vi "Read 3D Mesh Property Array.vi"(8 "error in (no error)":errorcluster, 11 "3D Mesh.lvclass in":refnum<class "3D Mesh.lvclass">) -> (0 "error out":errorcluster, 2 "3D Mesh Property Array":T1, 3 "3D Mesh.lvclass out":refnum<class "3D Mesh.lvclass">)   [LabVIEW 2020, in "3D Mesh.lvclass"]
uses:
  <vilib>/Math Plots/3D Math Plots/3D Mesh/3D Mesh/3D Mesh.lvclass
  <vilib>/Math Plots/3D Math Plots/3D Mesh/3D Mesh/Typedef/3D Mesh Propery Array.ctl
  <vilib>/Math Plots/3D Math Plots/3D Mesh/3D Mesh/Typedef/3D Mesh Property.ctl
  <vilib>/Math Plots/3D Math Plots/3D Plot/3D Plot/Typedef/Line Type.ctl
  <vilib>/Math Plots/3D Math Plots/3D Plot/3D Plot/Typedef/Color Ramp Cluster.ctl
  <vilib>/Math Plots/3D Math Plots/3D Mesh/3D Mesh/3D Mesh.lvclass/3D Mesh.ctl
  <vilib>/Math Plots/3D Math Plots/3D Plot/3D Plot/3D Plot.lvclass
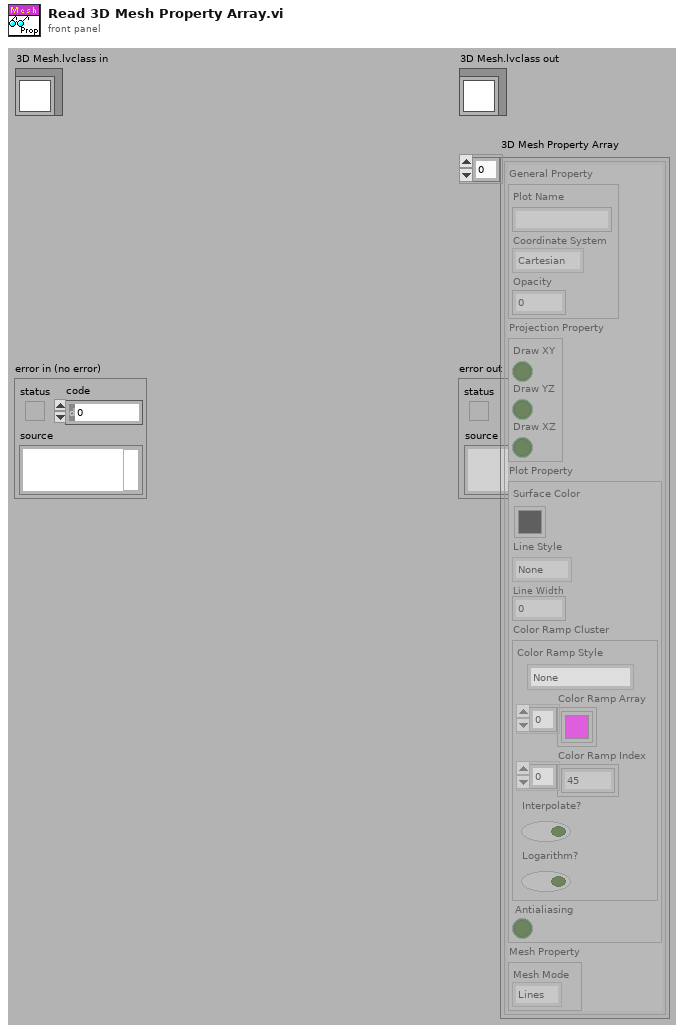
[diagram p1: front panel]
types:
  T1 = typedef "3D Mesh.lvclass/3D Mesh Propery Array.ctl" = T2[]
  T2 = typedef "3D Mesh.lvclass/3D Mesh Property.ctl" = cluster{"General Property":cluster{"Plot Name":string, "Coordinate System":enum16{"Cartesian", "Cylindrical", "Spherical"}, "Opacity":sgl}, "Projection Property":cluster{"Draw XY":bool, "Draw YZ":bool, "Draw XZ":bool}, "Plot Property":cluster{"Surface Color":u32, "Line Style":T3, "Line Width":sgl, "Color Ramp Cluster":T4, "Antialiasing":bool}, "Mesh Property":cluster{"Mesh Mode":enum16{"Lines", "Hidden Lines", "With Zero Plane"}}}
  T3 = typedef "3D Plot.lvclass/Line Type.ctl" = enum16{"None", "Solid", "Dash", "Dot", "Dash Dot"}
  T4 = typedef "3D Plot.lvclass/Color Ramp Cluster.ctl" = cluster{"Color Ramp Style":enum16{"None", "Shaded", "Color spectrum", "Grey scale", "Custom"}, "Color Ramp Array":u32[], "Color Ramp Index":i32[], "Interpolate?":bool, "Logarithm?":bool}
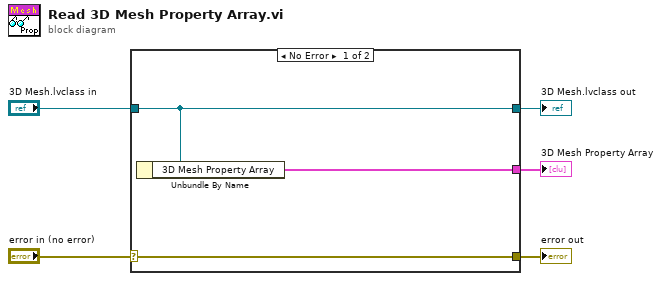
[diagram p0: block diagram]
diagram:
  n1 = case shown="No Error" "error in (no error)" {
    selector: "error in (no error)" -> [w8 w9]
    tunnel: [w8 w9] -> w4
    tunnel: [w7 w10] -> w2
    tunnel: "3D Mesh.lvclass in" -> [w7 w10]
    tunnel: [w6 _] -> w1
    frame No Error {
      n2 = Unbundle By Name(w7) -> ("3D Mesh Property Array"=w6:T1)
    }
    frame Error {
    }
  }
  "error out" <- w4
  "3D Mesh.lvclass out" <- w2
  "3D Mesh Property Array" <- w1
